vi "Get Velocity.vi"(8 "error in (no error)":errorcluster, 11 "KUKA youBot Arm Motor_EtherCAT in":refnum<class "NI_Robotics_KUKA youBot Arm Motor_EtherCAT.lvclass">) -> (0 "error out":errorcluster, 2 "CCW velocity (rpm)":dbl, 3 "KUKA youBot Arm Motor_EtherCAT out":refnum<class "NI_Robotics_KUKA youBot Arm Motor_EtherCAT.lvclass">)   [LabVIEW 2017, in "NI_Robotics_KUKA youBot Host.lvlib" / "NI_Robotics_KUKA youBot Arm Motor_EtherCAT.lvclass"]
uses:
  <vilib>/robotics/KUKA youBot/Motor/Arm Motor EtherCAT/NI_Robotics_KUKA youBot Arm Motor_EtherCAT.lvclass
  <vilib>/robotics/KUKA youBot/Motor/Arm Motor EtherCAT/NI_Robotics_KUKA youBot Arm Motor_EtherCAT.lvclass/NI_Robotics_KUKA youBot Arm Motor_EtherCAT.ctl
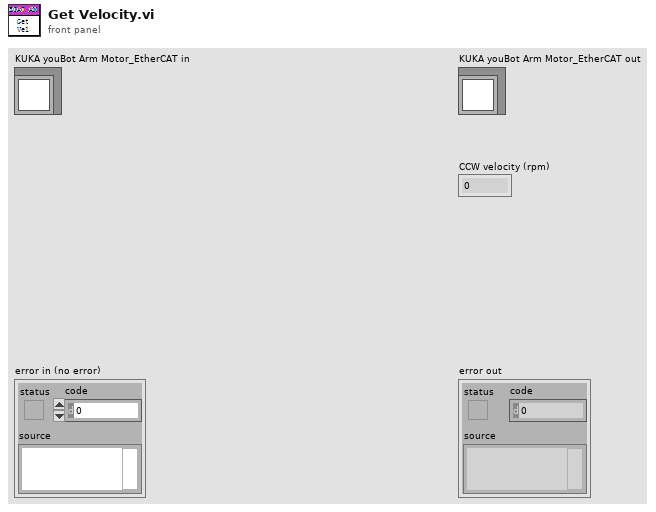
[diagram p1: front panel]
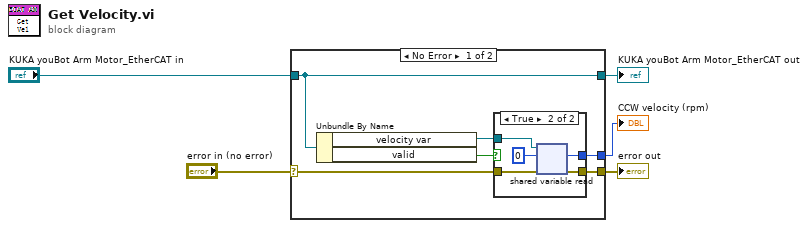
[diagram p0: block diagram]
diagram:
  n1 = case shown="No Error" "error in (no error)" {
    selector: "error in (no error)" -> [w10 w19]
    tunnel: "KUKA youBot Arm Motor_EtherCAT in" -> [w6 w18]
    tunnel: [w9 _] -> w3
    tunnel: [w8 w19] -> w2
    tunnel: [w6 w18] -> w1
    frame No Error {
      n2 = Unbundle By Name(w6) -> ("velocity var"=w11:refnum<k21>, "valid"=w7:bool)
      n3 = case shown="True" w7 {
        tunnel: w11 -> [_ w16]
        tunnel: w10 -> [w12 w15]
        tunnel: [_ w14] -> w9
        tunnel: [w12 w13] -> w8
        frame False {
        }
        frame True {
          n4 = shared-variable-read(w16, w15, 0 ("data type")) -> (w13:errorcluster, w14:i32)  [unwired: 2 out]
        }
      }
    }
    frame Error {
    }
  }
  "error out" <- w2
  "KUKA youBot Arm Motor_EtherCAT out" <- w1
  "CCW velocity (rpm)" <- w3
